vi "getRowColor.vi"(0 "reference in":refnum<class "Project Panels.lvclass">, 7 "Table in":refnum<vi>, 11 "error in (no error)":errorcluster) -> (4 "reference out":refnum<class "Project Panels.lvclass">, 15 "error out":errorcluster)   [LabVIEW 2015, in "Project Panels.lvclass"]
uses:
  Project Panels.lvclass
  APP/excelFile_class/fileType.ctl
  APP/excelFile_class/excelFile.lvclass
  SYS/File Controller_llb/File Controller.lvclass
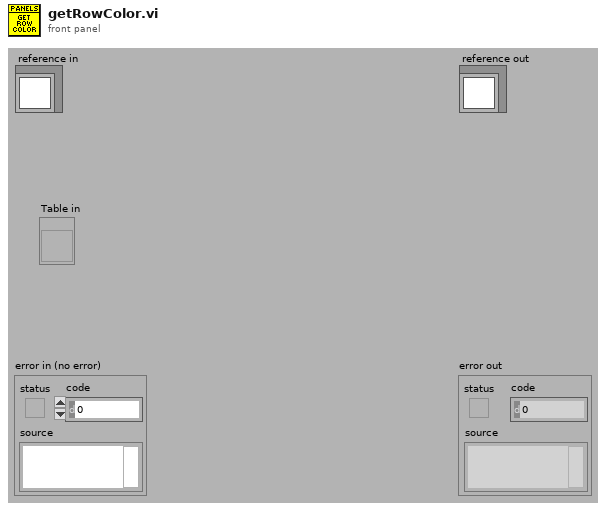
[diagram p1: front panel]
types:
  T1 = typedef "excelFile.lvclass/fileType.ctl" = enum16{"devices", "items", "partsTracking"}
  T2 = typedef "Project Panels.lvclass/ObjectAttributesRef.ctl" = refnum<data-value>
  T3 = typedef "Project Panels.lvclass/ObjectAttributes.ctl" = cluster{"MyAttribute":dbl, "device_controller_ref":refnum<class "Devices Controller.lvclass">, "file_controller_ref":refnum<class "File Controller.lvclass">, "item_controller_ref":refnum<class "Items Controller.lvclass">, "item_tables":cluster{"checkIN":string[][], "checkOUT":string[][], "storage":string[][]}, "quickbook_table":cluster{"notes":string[][]}, "notification_controller_ref":refnum<class "Notification Controller.lvclass">, "partstracking_controller_ref":refnum<class "PartsTracking Controller.lvclass">, "product_tables":cluster{"k4b2":string[][], "fitmate":string[][], "RMR":string[][], "CPET":string[][], "BP":string[][], "PP":string[][], "k5":string[][], "bb-pft":string[][]}, "rowsColour":u32[], "low_resolution?":bool}
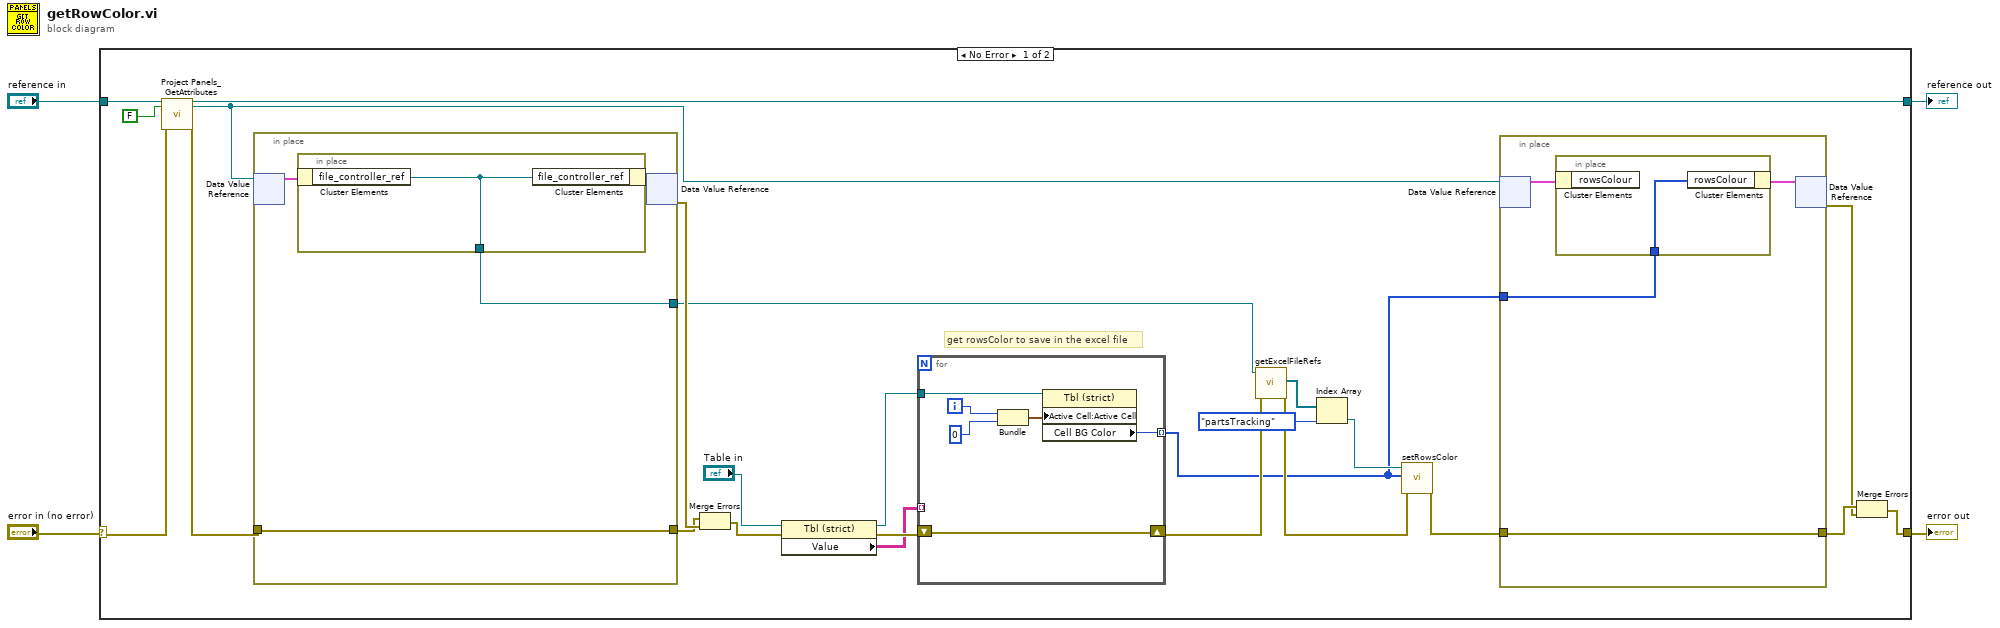
[diagram p0: block diagram]
diagram:
  n1 = case shown="No Error" "error in (no error)" {
    selector: "error in (no error)" -> [w24 w46]
    tunnel: [w7 w46] -> w3
    tunnel: [w22 w45] -> w1
    tunnel: "reference in" -> [w26 w45]
    frame No Error {
      # "get rowsColor to save in the excel file"
      n2 = call "Project Panels_GetAttributes.vi"("reference in"=w26, "return data? (T)"=FALSE, "error in (no error)"=w24) -> ("reference out"=w22:refnum<class "Project Panels.lvclass">, "attributes ref"=w5:T2, "error out"=w23:errorcluster)  [unwired: 13 in, 1 out]
      n3 = in-place {
        in-place-border: w23 -> [w41]
        in-place-border: [w41] -> w27
        in-place-border: [w40] -> w11
        n4 = in-place-dvr #1(w5) -> (w42:T3)  [unwired: 1 out]
        n5 = in-place {
          in-place-border: [w44] -> w40
          n6 = in-place-cluster #2(w42) -> ("file_controller_ref"=w44:refnum<class "File Controller.lvclass">)
          n7 = in-place-cluster #2("file_controller_ref"=w44) -> (w43:T3)
        }
        n8 = in-place-dvr #1(w43) -> (w28:errorcluster)  [unwired: 1 out]
      }
      n9 = Merge Errors(w27, w28) -> (w13:errorcluster)
      n10 = property on="Property Node" class="Tbl (strict)"(reference="Table in", error in=w13) -> (reference out=w14:refnum<vi>, error out=w21:errorcluster, "Value"=w15:string[][])
      n11 = for {
        shift-right: [w39] -> w19
        shift-left: w21 -> [w39]
        tunnel: w15 -> [_] mode=indexing
        tunnel: w14 -> [w35]
        tunnel: [w34] -> w6 mode=indexing
        i -> [w38]
        n12 = Bundle(w38, 0) -> (w36:cluster{i32, i32})  [unwired: 1 in]
        n13 = property on="Property Node" class="Tbl (strict)"(reference=w35, "Active Cell:Active Cell"=w36) -> ("Cell BG Color"=w34:u32)  [unwired: 1 in, 2 out]
      }
      n14 = call "getExcelFileRefs.vi"("error in (no error)"=w19, "reference in"=w11) -> ("error out"=w18:errorcluster, "excelFile_refs"=w20:refnum<class "excelFile.lvclass">[])  [unwired: 7 in, 1 out]
      n15 = Index Array(array=w20, index=fileType."partsTracking" ("fileType")) -> (element=w16:refnum<class "excelFile.lvclass">)
      n16 = call "setRowsColor.vi"("error in (no error)"=w18, "rowsColor"=w6, "reference in"=w16) -> ("error out"=w10:errorcluster)  [unwired: 7 in, 1 out]
      n17 = in-place {
        in-place-border: w10 -> [w30]
        in-place-border: [w30] -> w9
        in-place-border: w6 -> [w29]
        n18 = in-place-dvr #3(w5) -> (w31:T3)  [unwired: 1 out]
        n19 = in-place {
          in-place-border: w29 -> [w33]
          n20 = in-place-cluster #4(w31) -> ()  [unwired: 1 out]
          n21 = in-place-cluster #4("rowsColour"=w33) -> (w32:T3)
        }
        n22 = in-place-dvr #3(w32) -> (w8:errorcluster)  [unwired: 1 out]
      }
      n23 = Merge Errors(w9, w8) -> (w7:errorcluster)
    }
    frame Error {
    }
  }
  "error out" <- w3
  "reference out" <- w1
